vi "tm_waitnextframe.vi"(8 "error in (no error)":errorcluster, 10 "Timeout":i32=5000, 11 "Handle in":u32) -> (0 "error out":errorcluster, 1 "Frame Count":i32, 2 "Frame Index":i32, 3 "Handle out":u32)   [LabVIEW 2015]
uses:
  tmcamcon.dll
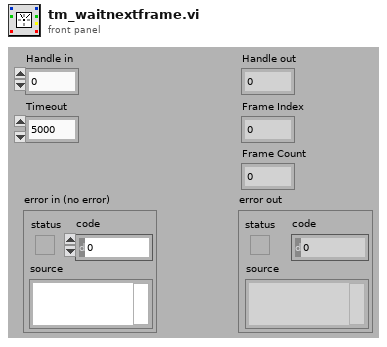
[diagram p1: front panel]
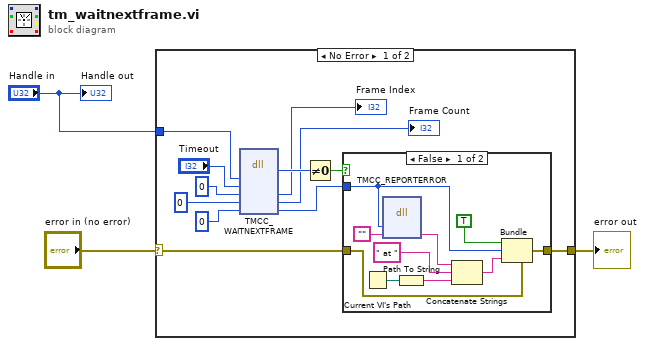
[diagram p0: block diagram]
diagram:
  n1 = case shown="No Error" "error in (no error)" {
    selector: "error in (no error)" -> [w11 w27]
    tunnel: [w10 w27] -> w2
    tunnel: "Handle in" -> [w8 _]
    frame No Error {
      n2 = dll-call lib="tmcamcon.dll" fn="TMCC_WAITNEXTFRAME"("HDCAM"=w8, "timeout"="Timeout", "frameindex"=0 ("Erval"), "framecount"=0 ("Erval"), "Erval"=0) -> ("return type"=w15:u32, "frameindex"=→"Frame Index":i32, "framecount"=→"Frame Count":i32, "Erval"=w12:i32)  [unwired: 5 in, 2 out]
      n3 = Not Equal To 0?(x=w15) -> (x != 0?=w13:bool)
      n4 = case shown="False" w13 {
        tunnel: w11 -> [w25 w26]
        tunnel: [w24 w26] -> w10
        tunnel: w12 -> [w18 _]
        frame False {
          n5 = Current VI's Path() -> (path=w23:path)
          n6 = dll-call lib="tmcamcon.dll" fn="TMCC_REPORTERROR"("error"=w18, "buf"="") -> ("buf"=w17:string)  [unwired: 5 in, 2 out]
          n7 = Path To String(path=w23) -> (string=w19:string)
          n8 = Concatenate Strings(w17, " at ", w19) -> (w22:string)
          n9 = Bundle(cluster=w25, "status"=TRUE, "code"=w18, "source"=w22) -> (w24:errorcluster)
        }
        frame True {
        }
      }
    }
    frame Error {
    }
  }
  "error out" <- w2
  "Handle out" <- "Handle in"
